vi "VISA Read With CSMLog(Hex).vi"(7 "Place(\"\" to use VI's Name)":string, 8 "error in (no error)":errorcluster, 10 "byte count":u32, 11 "VISA Refnum in":refnum<visa-resource-name>) -> (0 "error out":errorcluster, 2 "read buffer":string, 3 "VISA Refnum out":refnum<visa-resource-name>)   [LabVIEW 2020]
uses:
  <userlib>/_NEVSTOP/Communicable State Machine(CSM)/AdvanceAPI/CSM - Convert Error to Argument.vi
  <userlib>/_NEVSTOP/Communicable State Machine(CSM)/AdvanceAPI/CSM - Make String Arguments Safe.vi
  <userlib>/_NEVSTOP/Communicable State Machine(CSM)/AdvanceAPI/CSM - Keywords.vi
  <userlib>/_NEVSTOP/Communicable State Machine(CSM)/_Support/GlobalEvent/FGV-GlobalEventRef.vi
  <userlib>/_NEVSTOP/Communicable State Machine(CSM)/Communicable State Machine.lvlib
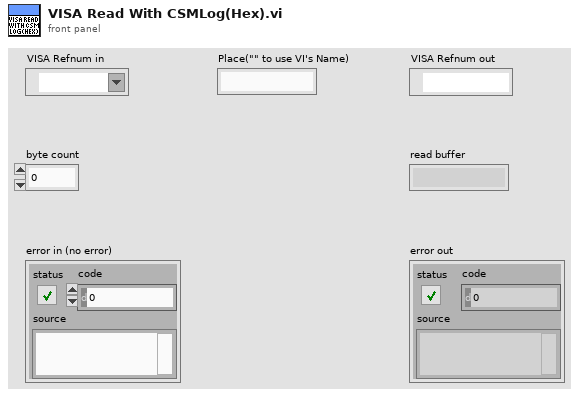
[diagram p1: front panel]
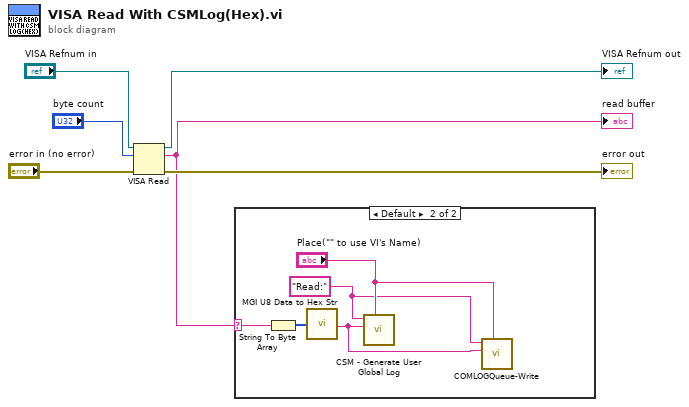
[diagram p0: block diagram]
diagram:
  n1 = VISA Read(VISA resource name="VISA Refnum in", byte count="byte count", error in (no error)="error in (no error)") -> (VISA resource name out=→"VISA Refnum out":refnum<visa-resource-name>, read buffer=w1:string, error out=→"error out":errorcluster)  [unwired: 1 out]
  "read buffer" <- w1
  n2 = case shown="Default" w1 {
    selector: w1 -> [_ w10]
    frame "" {
    }
    frame Default {
      w8 = "Read:" ("Log")
      n3 = String To Byte Array(string=w10) -> (unsigned byte array=w11:u8[])
      n4 = call <userlib>:"MGI U8 Data to Hex Str.vi"("u8 Data[]"=w11) -> ("HEX String (0-9,A-F)"=w7:string)
      n5 = call <userlib>:"CSM - Generate User Global Log.vi"("Place(\"\" to use VI's Name)"="Place(\"\" to use VI's Name)", "Arguments"=w7, "Log"=w8) -> ()  [unwired: 8 in, 1 out]
      n6 = call "COMLOGQueue-Write.vi"("COM(Constant)"="Place(\"\" to use VI's Name)", "element"=w7, "Prefix"=w8) -> ()  [unwired: 6 in, 1 out]
    }
  }
